vi "CheckforChange.vi"(8 "error in (no error)":errorcluster, 11 "OnChange_Boolean in":refnum<class "OnChangeNotifier_I64.lvclass">) -> (0 "error out":errorcluster, 3 "OnChange_Boolean out":refnum<class "OnChangeNotifier_I64.lvclass">)   [LabVIEW 2021, in "OnChangeNotifier_I64.lvclass"]
uses:
  OnChangeNotifier_I64.lvclass
  <vilib>/TSA/Abstract Data Classes/Abs_Types/I32 Integer/Static Read.vi
  <vilib>/TSA/Abstract Data Classes/Abs_Types/I32 Integer/Abs_I32 Integer.lvclass
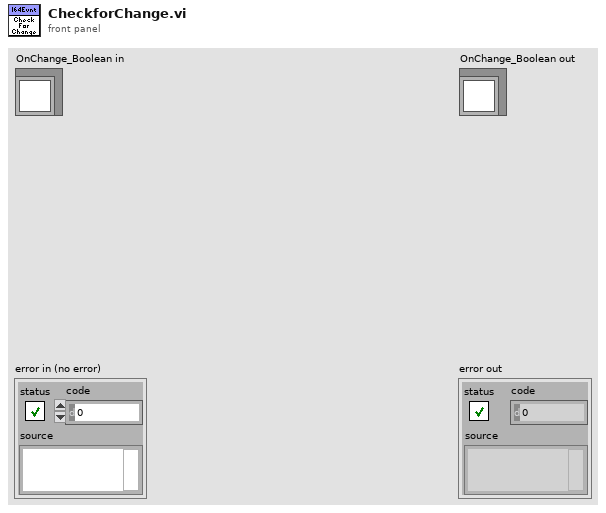
[diagram p1: front panel]
types:
  T1 = typedef "OnChangeNotifier_I64.lvclass/Class Type.ctl" = refnum<class "Abs_I32 Integer.lvclass">
  T2 = typedef "OnChangeNotifier_I64.lvclass/Type.ctl" = i32
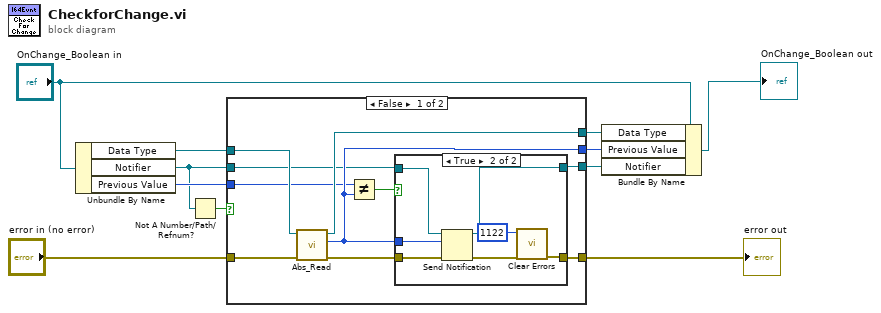
[diagram p0: block diagram]
diagram:
  n1 = Unbundle By Name("OnChange_Boolean in") -> ("Data Type"=w11:T1, "Notifier"=w1:refnum<notifier>, "Previous Value"=w3:T2)
  n2 = Not A Number/Path/Refnum?(number/path/refnum=w1) -> (NaN/Path/Refnum?=w2:bool)
  n3 = case shown="False" w2 {
    tunnel: w11 -> [w21 w31]
    tunnel: [w20 w31] -> w10
    tunnel: "error in (no error)" -> [w19 w34]
    tunnel: [w17 w32] -> w6
    tunnel: w1 -> [w16 w33]
    tunnel: [w15 w33] -> w5
    tunnel: [w14 w34] -> w4
    tunnel: w3 -> [w12 w32]
    frame False {
      n4 = call-poly <vilib>:"Abs_Read.vi"("error in (no error)"=w19, "Abs_I32 Integer in"=w21) -> ("error out"=w18:errorcluster, "Value"=w17:i32, "Abs_I32 Integer out"=w20:T1)  [unwired: 7 in]
      n5 = Not Equal?(x=w12, y=w17) -> (x != y?=w13:bool)
      n6 = case shown="True" w13 {
        tunnel: w18 -> [w22 w29]
        tunnel: w17 -> [_ w27]
        tunnel: w16 -> [w23 w30]
        tunnel: [w23 w28] -> w15
        tunnel: [w22 w26] -> w14
        frame False {
        }
        frame True {
          n7 = Send Notification(notification=w27, notifier=w30, error in (no error)=w29) -> (notifier out=w28:refnum<notifier>, error out=w25:errorcluster)
          n8 = call <vilib>:"Clear Errors.vi"("error in (no error)"=w25, "specific error code to clear (0: all)"=1122) -> ("error out"=w26:errorcluster)  [unwired: 4 in, 1 out]
        }
      }
    }
    frame True {
    }
  }
  "error out" <- w4
  n9 = Bundle By Name(cluster="OnChange_Boolean in", "Data Type"=w10, "Previous Value"=w6, "Notifier"=w5) -> (→"OnChange_Boolean out":refnum<class "OnChangeNotifier_I64.lvclass">)
